vi "SMSMagnet.i attribute.vi"(0 "VI Refnum":refnum<vi>, 2 "CLASS.i attribute":T1, 3 "Action":T3(ring), 5 "error in (no error)":errorcluster) -> (14 "VI Refnum out":refnum<vi>, 16 "CLASS.i attribute out":T1, 19 "error out":errorcluster)   [LabVIEW 2014, in "SMSMagnet.lvlib"]
doc: "This is a so-called functional global variable. It manages the access to a global variable in a thread-safe way. \n\nHere the attribute data of all instances of THIS class are stored. This is done for performance reasons.\n\nLicense Agreement for this software:\n\nCopyright (C)\nGesellschaft für Schwerionenforschung, GSI\nPlanckstr. 1\n64291 Darmstadt\nGermany\n\nContact: D.Beck@gsi.de \n\nThis program is free software; you can redistribute it and/or modify it under the terms of the GNU General Public License as published by the Free Software Foundation; either version 2 of the license, or (at your option) any later version.\n\nThis program is distributed in the hope that it will be useful, but WITHOUT ANY WARRANTY; without even the implied warranty of MERCHANTABILITY or FITNESS FOR A PARTICULAR PURPOSE. See the GNU General License for more details (http://www.gnu.org).\n\nGesellschaft für Schwerionenforschung, GSI\nPlanckstr. 1, 64291 Darmstadt, Germany\nFor all questions and ideas contact: M.Richter@gsi.de, H.Brand@gsi.de or D.Beck@gsi.de.\nLast update: 17-JUN-2004"
uses:
  SMSMagnet.lvlib
  SMSMagnet.i attribute.ctl
  CS_Core/CSSystem/CoreDefs/CoreDefs.error_type.ctl
  CS_Core/CSSystem/CoreLib/CoreLib.lvlib
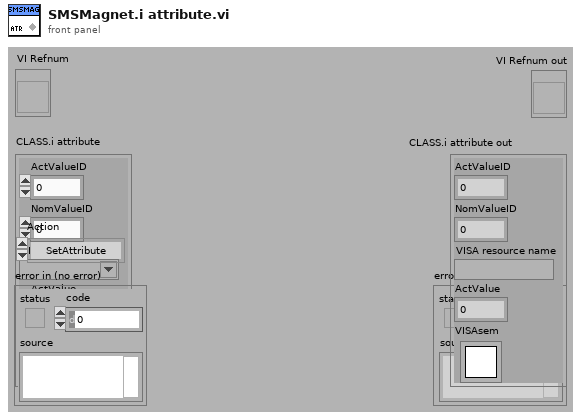
[diagram p1: front panel]
types:
  T1 = typedef "SMSMagnet.lvlib/SMSMagnet.i attribute.ctl" = cluster{"ActValueID":i32, "NomValueID":i32, "VISA resource name":refnum<visa-resource-name>, "ActValue":dbl, "VISAsem":T2}
  T2 = typedef "Semaphore RefNum" = refnum<k1>
  T3 = enum16{"SetAttribute", "GetAttribute", "CreateAttribute", "DestroyAttribute", "DestroyAllAtributes"}
  T4 = typedef "CoreDefs.error_type.ctl" = enum16{"no error", "can't load process", "can't unload process", "process does not exist", "can't install process", "can't remove process", "unknown function", "time out", "can't execute function", "duplicate queue name", "super not found", "caller queue invalid", "can't ping process", "unknown error", "VISA Error", "VISA timeout", "GPIB timeout", "GPIB error", "communication error", "data type mismatch", "can't read data from OPC server", "can't write data to OPC server", "OET error", "function not implemented", "process already exists", "invalid Shared Variable name", "error writing Shared Variable", "error reading Shared Variable", "invalid client name", "corrupt database", "unknown class", "call not authorized", "parameter out of range", "OET timeout: can't get data to modify", "invalid queue name", "requested operation incompatible with current state", "event undefined", "event disabled", "state undefined", "caller is not a friend", "EventBuilder: bad eventID", "EventBuilder: no DAQ devices", "a thread must not stop itself", "UNUSED ELEMENT4", "DiscArchiver: eventData incomplete", "DiscArchiver: eventData does not belong to run", "DiscArchiver: can't open file", "DiscArchiver: can't write to file", "DiscArchiver: available disc space low", "can't acquire semaphore", "error reading data from database", "notifier object is not existing", "can't register process", "can't unregister process", "illegal event type", "object disabled", "object already exists", "can't change state", "Instrument not found", "no connection to remote node", "invalid reference", "N/A", "UNUSED ELEMENT 1", "element not found", "illegal TCP/IP connection detected", "object does not exist", "invalid access ID", "unknown CS system", "invalid privilige", "unsupported data type", "unsupported server type", "IO server already exists", "Shared Variable already exists"}
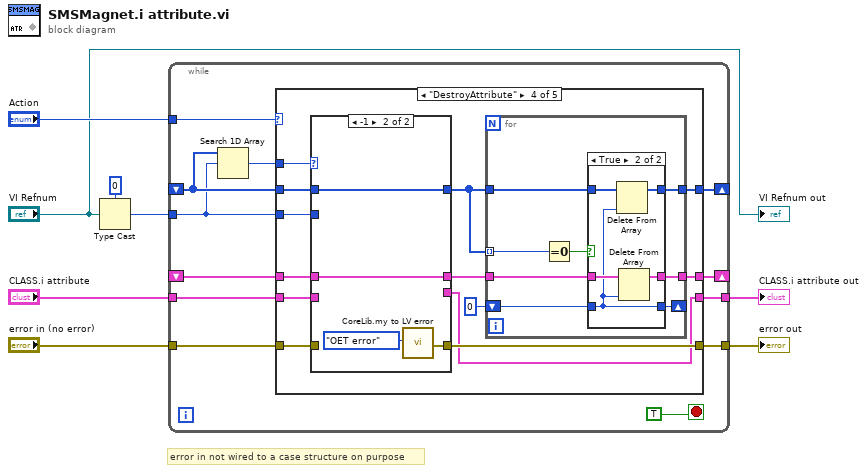
[diagram p0: block diagram]
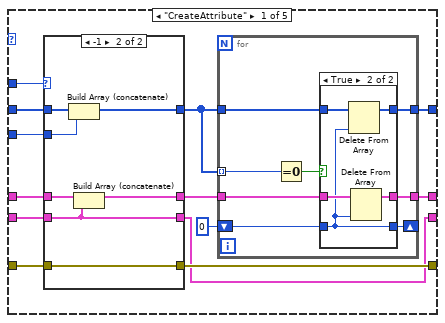
[diagram p2: hidden frame]
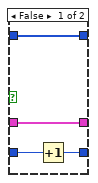
[diagram p3: hidden frame]
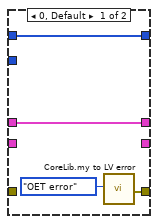
[diagram p4: hidden frame]
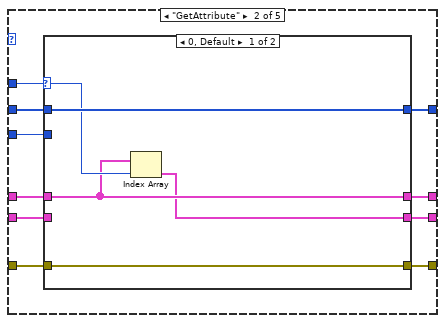
[diagram p5: hidden frame]
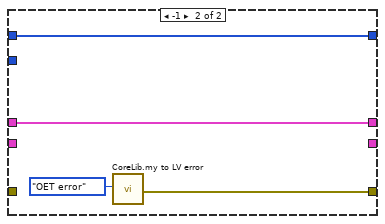
[diagram p6: hidden frame]
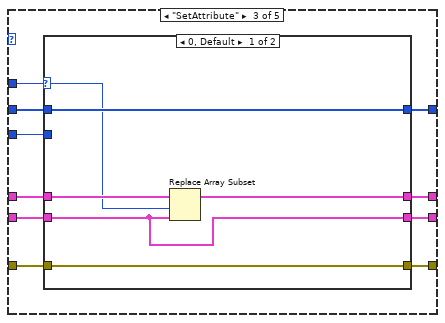
[diagram p7: hidden frame]
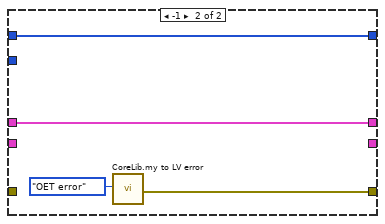
[diagram p8: hidden frame]
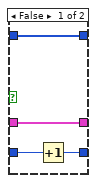
[diagram p9: hidden frame]
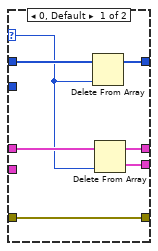
[diagram p10: hidden frame]
diagram:
  # "error in not wired to a case structure on purpose"
  n1 = Type Cast(type=0, x="VI Refnum") -> (*(type *) &x=w1:i32)
  n2 = while {
    shift-right: [w14] -> _
    shift-left: _ -> [w15]
    tunnel: "Action" -> [w19]
    shift-right: [w16] -> _
    shift-left: _ -> [w12]
    tunnel: w1 -> [w11]
    tunnel: "error in (no error)" -> [w18]
    tunnel: [w17] -> w6
    tunnel: "CLASS.i attribute" -> [w13]
    tunnel: [w9] -> w4
    stop <- TRUE stop-if-true
    n3 = Search 1D Array(1D array=w12, element=w11) -> (index of element=w10:i32)  [unwired: 1 in]
    n4 = case shown="\"DestroyAttribute\"" w19 {
      tunnel: w12 -> [w31 w69 w88 w111 _]
      tunnel: w11 -> [w30 w67 w86 w110 _]
      tunnel: w18 -> [w33 w71 w90 w113 w142]
      tunnel: [w32 w70 w89 w112 w142] -> w17
      tunnel: [w25 w68 w87 w105 _] -> w16
      tunnel: w15 -> [w29 w66 w85 w109 _]
      tunnel: [w24 w65 w84 w103 _] -> w14
      tunnel: w13 -> [w28 w64 w83 w108 _]
      tunnel: w10 -> [w27 w63 w82 w107 _]
      tunnel: [w21 w62 w81 w101 _] -> w9
      frame "CreateAttribute" {
        n5 = case shown="-1" w27 {
          tunnel: w33 -> [_ w61]
          tunnel: [w53 w61] -> w32
          tunnel: w31 -> [w52 w60]
          tunnel: [w52 w59] -> w23
          tunnel: w30 -> [_ w58]
          tunnel: w29 -> [w51 w57]
          tunnel: [w51 w56] -> w22
          tunnel: w28 -> [_ w55]
          tunnel: [_ w55] -> w21
          frame 0, Default {
            n6 = call "CoreLib.my to LV error.vi"("ErrorTypes"=CoreDefs.error_type."OET error") -> ("myErrorCluster"=w53:errorcluster)  [unwired: 17 in, 1 out]
          }
          frame -1 {
            n7 = Build Array (concatenate)(w60, w58) -> (w59:i32[])
            n8 = Build Array (concatenate)(w57, w55) -> (w56:T1[])
          }
        }
        n9 = for {
          tunnel: w23 -> [w38]
          tunnel: [w37] -> w25
          tunnel: [w41] -> w24
          tunnel: w22 -> [w40]
          tunnel: w23 -> [w36] mode=indexing
          shift-right: [w35] -> _
          shift-left: 0 -> [w34]
          n10 = Equal To 0?(x=w36) -> (x = 0?=w39:bool)
          n11 = case shown="True" w39 {
            tunnel: [w45 w50] -> w41
            tunnel: w40 -> [w45 w49]
            tunnel: [w44 w47] -> w37
            tunnel: w38 -> [w44 w48]
            tunnel: w34 -> [w43 w46]
            tunnel: [w42 w46] -> w35
            frame False {
              n12 = Increment(x=w43) -> (x+1=w42:i32)
            }
            frame True {
              n13 = Delete From Array(array=w48, index=w46) -> (array with subset deleted=w47:i32[])  [unwired: 1 in, 1 out]
              n14 = Delete From Array(array=w49, index=w46) -> (array with subset deleted=w50:T1[])  [unwired: 1 in, 1 out]
            }
          }
        }
      }
      frame "GetAttribute" {
        n15 = case shown="0, Default" w63 {
          selector: w63 -> [w74 _]
          tunnel: w71 -> [w76 _]
          tunnel: [w76 w79] -> w70
          tunnel: w69 -> [w75 w78]
          tunnel: [w75 w78] -> w68
          tunnel: w67 -> [_ _]
          tunnel: w66 -> [w73 w77]
          tunnel: [w73 w77] -> w65
          tunnel: w64 -> [_ _]
          tunnel: [w72 _] -> w62
          frame 0, Default {
            n16 = Index Array(array=w73, index=w74) -> (element=w72:T1)
          }
          frame -1 {
            n17 = call "CoreLib.my to LV error.vi"("ErrorTypes"=CoreDefs.error_type."OET error") -> ("myErrorCluster"=w79:errorcluster)  [unwired: 17 in, 1 out]
          }
        }
      }
      frame "SetAttribute" {
        n18 = case shown="0, Default" w82 {
          selector: w82 -> [w92 _]
          tunnel: w90 -> [w96 _]
          tunnel: [w96 w99] -> w89
          tunnel: w88 -> [w95 w98]
          tunnel: [w95 w98] -> w87
          tunnel: w86 -> [_ _]
          tunnel: w85 -> [w94 w97]
          tunnel: [w93 w97] -> w84
          tunnel: w83 -> [w91 _]
          tunnel: [w91 _] -> w81
          frame 0, Default {
            n19 = Replace Array Subset(array=w94, new element=w91, index=w92) -> (w93:T1[])
          }
          frame -1 {
            n20 = call "CoreLib.my to LV error.vi"("ErrorTypes"=CoreDefs.error_type."OET error") -> ("myErrorCluster"=w99:errorcluster)  [unwired: 17 in, 1 out]
          }
        }
      }
      frame "DestroyAttribute" {
        n21 = case shown="-1" w107 {
          selector: w107 -> [w133 _]
          tunnel: w113 -> [w137 _]
          tunnel: [w137 w140] -> w112
          tunnel: w111 -> [w136 w139]
          tunnel: [w135 w139] -> w104
          tunnel: w110 -> [_ _]
          tunnel: w109 -> [w134 w138]
          tunnel: [w132 w138] -> w102
          tunnel: w108 -> [_ _]
          tunnel: [w131 _] -> w101
          frame 0, Default {
            n22 = Delete From Array(array=w136, index=w133) -> (array with subset deleted=w135:i32[])  [unwired: 1 in, 1 out]
            n23 = Delete From Array(array=w134, index=w133) -> (deleted portion=w131:T1, array with subset deleted=w132:T1[])  [unwired: 1 in]
          }
          frame -1 {
            n24 = call "CoreLib.my to LV error.vi"("ErrorTypes"=CoreDefs.error_type."OET error") -> ("myErrorCluster"=w140:errorcluster)  [unwired: 17 in, 1 out]
          }
        }
        n25 = for {
          tunnel: w104 -> [w118]
          tunnel: [w117] -> w105
          tunnel: [w121] -> w103
          tunnel: w102 -> [w120]
          tunnel: w104 -> [w116] mode=indexing
          shift-right: [w115] -> _
          shift-left: 0 -> [w114]
          n26 = Equal To 0?(x=w116) -> (x = 0?=w119:bool)
          n27 = case shown="True" w119 {
            tunnel: [w125 w130] -> w121
            tunnel: w120 -> [w125 w129]
            tunnel: [w124 w127] -> w117
            tunnel: w118 -> [w124 w128]
            tunnel: w114 -> [w123 w126]
            tunnel: [w122 w126] -> w115
            frame False {
              n28 = Increment(x=w123) -> (x+1=w122:i32)
            }
            frame True {
              n29 = Delete From Array(array=w128, index=w126) -> (array with subset deleted=w127:i32[])  [unwired: 1 in, 1 out]
              n30 = Delete From Array(array=w129, index=w126) -> (array with subset deleted=w130:T1[])  [unwired: 1 in, 1 out]
            }
          }
        }
      }
      frame "DestroyAllAtributes" {
      }
    }
  }
  "error out" <- w6
  "CLASS.i attribute out" <- w4
  "VI Refnum out" <- "VI Refnum"
